vi "Configure Output On Off.vi"(7 "Slave Address":i32=-1 min=-1 max=30 step=1, 8 "error":errorcluster, 9 "Settle (0 mS)":u32, 10 "Output ON":bool, 11 "VISA":refnum<visa-resource-name>) -> (0 "error out":errorcluster, 3 "VISA out":refnum<visa-resource-name>)   [LabVIEW 2019, in "TDK-Lambda GEN LAN Series.lvlib"]
doc: "Configure the power supply output ON or OFF. No other settings change.\nIf \"Output ON\" is set FALSE, the output will be turned OFF.\n\nThis VI will wait for \"Settle\" milliseconds after setting the output. If unwired, there will be no delay"
uses:
  <instrlib>/TDK-Lambda GEN LAN Series/TDK-Lambda GEN LAN Series.lvlib
panel:
  # "TDK-Lambda Genesys \n  LAN\n  DC Power Supplies"
  # "Set Output ON or OFF"
  # "(c) 2019 TDK-Lambda.  ALL RIGHTS RESERVED."
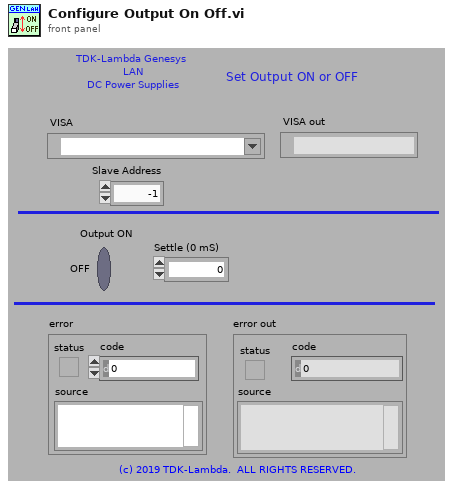
[diagram p1: front panel]
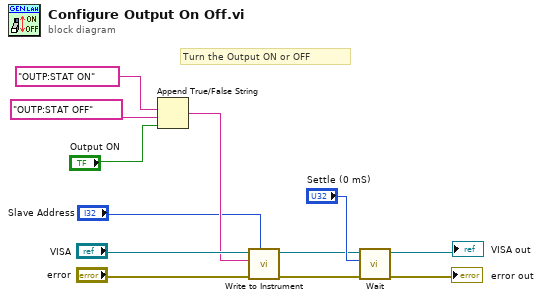
[diagram p0: block diagram]
diagram:
  # "Turn the Output ON or OFF"
  n1 = Append True/False String(1:"Output ON", 2:"OUTP:STAT OFF" ("format string"), 3:"OUTP:STAT ON" ("format string")) -> (0:w4:string)  [unwired: 1 in]
  n2 = call <instrlib>:"Write to Instrument.vi"("Slave Address"="Slave Address", "error"="error", "Command"=w4, "VISA"="VISA") -> ("error out"=w8:errorcluster, "VISA out"=w7:refnum<visa-resource-name>)  [unwired: 6 in]
  n3 = call <instrlib>:"Wait.vi"("error"=w8, "Delay (20 mS)"="Settle (0 mS)", "VISA"=w7) -> ("error out"=→"error out":errorcluster, "VISA out"=→"VISA out":refnum<visa-resource-name>)  [unwired: 7 in]
